vi "Tektronix TDS 200 1000 2000 Series Acquire Trend Plot.vi"() -> ()   [LabVIEW 2012]
doc: "This example shows how to acquire the trend plot data.\n\n<b>Note(s):</b>\nThis Example is only applicable for TBS1000B series models."
uses:
  <instrlib>/Tektronix TDS 200 1000 2000 Series/Tektronix TDS 200 1000 2000 Series.lvlib
panel:
  out "Elapsed Time":string
  in  "Trend Plot Type (0: Frequency)":i32(ring) items=["None", "Phase", "DelayRR", "DelayRF", "DelayFR", "DelayFF", "Frequency", "Mean", "Period", "Positive Duty", "Negative Duty", "Peak to Peak", "Cycle RMS", "Minimum", "Maximum", "Rise Time", "Fall Time", "Positive Width", "Negative Width", "Amplitude", "Cycle Mean", "High", "Low", "Positive Overshoot", "Negative Overshoot", "Cursor Mean", "Burst Width", "Positive Pulse Count", "Negative Pulse Count", "Rising Edge Count", "Falling Edge Count", "Area", "Cycle Area", "RMS", "Cursor RMS"]
  out "Scale":dbl
  out "Maximum Scale":dbl
  out "Minimum Scale":dbl
  out "Maximum Value":dbl
  out "Minimum Value":dbl
  out "Average Value":dbl
  out "Units":string
  in  "Channel Number (1: Trend Plot 1)":i32(ring)=1 items=["Trend Plot 1"=1, "Trend Plot 2"=2]
  in  "Trend Plot Source (0: Channel 1)":i32(ring) items=["Channel 1", "Channel 2", "Math", "Channel 1 - Channel 2", "Channel 2 - Channel 1", "Channel 1 - Math", "Math - Channel 1", "Channel 2-Math", "Math - Channel 2"]
  in  "Serial Configuration":T1={"Baud Rate"=9600, "Parity"=0, "Stop Bits"=10, "Flow Control"=2} {"Flow Control" items=["None", "XON/XOFF", "RTS/CTS", "XON/XOFF & RTS/CTS", "DTR/DSR", "XON/XOFF & DTR/DSR"]; "Stop Bits" items=["1.0"=10, "1.5"=15, "2.0"=20]; "Parity" items=["None", "Odd", "Even", "Mark", "Space"]; "Baud Rate" items=["300"=300, "600"=600, "1200"=1200, "2400"=2400, "4800"=4800, "9600"=9600, "19200"=19200]}
  in  "VISA resource name":refnum<visa-resource-name>
  # "(C) 2009-2014 National Instruments.  ALL RIGHTS RESERVED."
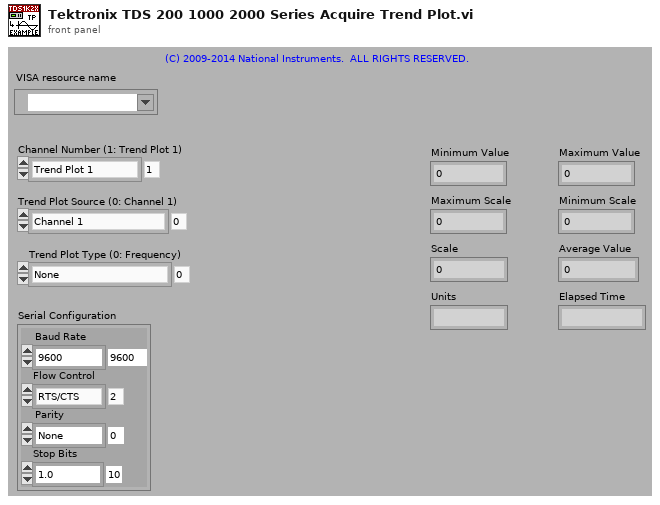
[diagram p1: front panel]
types:
  T1 = cluster{"Baud Rate":u32, "Parity":u16, "Stop Bits":u16, "Flow Control":u16}
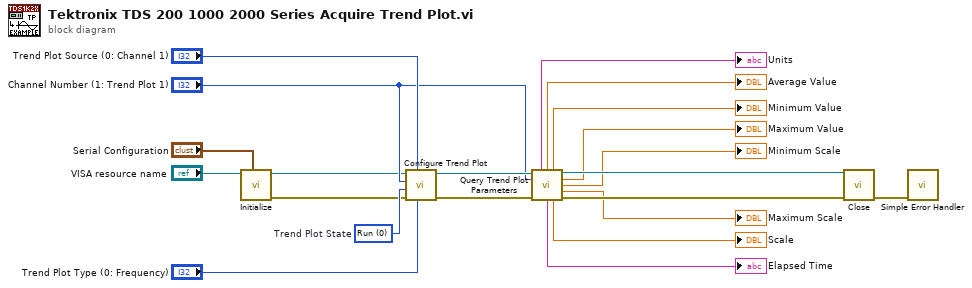
[diagram p0: block diagram]
diagram:
  w15 = 0 items=["Run", "Stop"]  # Trend Plot State
  n1 = call <instrlib>:"Initialize.vi"("Serial Configuration"="Serial Configuration", "VISA resource name"="VISA resource name") -> ("error out"=w3:errorcluster, "VISA resource name out"=w4:refnum<visa-resource-name>)  [unwired: 3 in, 5 out]
  n2 = call <instrlib>:"Configure Trend Plot.vi"("Trend Plot Type (0: Frequency)"="Trend Plot Type (0: Frequency)", "Trend Plot Source (0: Channel 1)"="Trend Plot Source (0: Channel 1)", "error in (no error)"=w3, "Trend Plot State (0: Run)"=w15, "Channel Number (1: Trend Plot 1)"="Channel Number (1: Trend Plot 1)", "VISA resource name"=w4) -> ("error out"=w17:errorcluster, "VISA resource name out"=w18:refnum<visa-resource-name>)  [unwired: 4 out]
  n3 = call <instrlib>:"Query Trend Plot Parameters.vi"("VISA resource name"=w18, "Channel Number (1: Trend Plot 1)"="Channel Number (1: Trend Plot 1)", "error in (no error)"=w17) -> ("Units"=→"Units":string, "Average Value"=→"Average Value":dbl, "Minimum Value"=→"Minimum Value":dbl, "VISA resource name out"=w14:refnum<visa-resource-name>, "Maximum Value"=→"Maximum Value":dbl, "Minimum Scale"=→"Minimum Scale":dbl, "Maximum Scale"=→"Maximum Scale":dbl, "Elapsed Time"=→"Elapsed Time":string, "Scale"=→"Scale":dbl, "error out"=w13:errorcluster)  [unwired: 3 in]
  n4 = call <instrlib>:"Close.vi"("error in (no error)"=w13, "VISA resource name"=w14) -> ("error out"=w21:errorcluster)  [unwired: 9 out]
  n5 = call <vilib>:"Simple Error Handler.vi"("error in (no error)"=w21) -> ()  [unwired: 1 in, 8 out]
